vi "Dispatch PVMonitors.vi"(8 "Error In":errorcluster, 10 "PV Names (empty)":string[](array[string]), 11 "CS++GUIActor in":refnum<class "CS++GUIActor.lvclass">) -> (0 "Error Out":errorcluster, 3 "CS++GUIActor out":refnum<class "CS++GUIActor.lvclass">)   [LabVIEW 2015, in "CS++GUIActor.lvlib" / "CS++GUIActor.lvclass"]
doc: "Dispatch nested PVMonitor actors according to PV protocoll prefix."
uses:
  CS++GUIActor.lvclass
  CS++GUIActor Messages/Update-PV Msg/Update-PV Msg.lvclass
  CS++PVMonitor/CS++PVMonitor.lvclass
  CS++PVMonitor Messages/CS++PVUpdate Msg/CS++PVUpdate Msg.lvclass/CS++PVUpdate Msg.ctl
  CS++BaseActor/CS++BaseActor.lvclass/CS++BaseActor.ctl
  CS++GUIActor.lvclass/CS++GUIActor.ctl
  <vilib>/ActorFramework/Actor/Actor.lvclass/Actor.ctl
  <vilib>/ActorFramework/Message Enqueuer/Message Enqueuer.lvclass/Message Enqueuer.ctl
  Classes/CS++ProcessVariables/ProcessVariable/PV.lvclass/PV.ctl
  CS++PVMonitor/CS++PVMonitor.lvclass/CS++PVMonitor.ctl
  CS++PVMonitor Messages/Register PVs Msg/Register PVs Msg.lvclass/Register PVs Msg.ctl
  CS++BaseActor/Read Object Name.vi
  CS++BaseActor/Read CS++Factory.vi
  Read Associated Actor Name.vi
  <vilib>/ActorFramework/Message Enqueuer/Init from Existing Queue.vi
  <vilib>/ActorFramework/Message Enqueuer/Enqueue.vi
  <vilib>/ActorFramework/Message Priority Queue/Priority Enqueue.vi
  Classes/CS++ProcessVariables/ProcessVariable/PV.lvclass
  Classes/CS++BaseClasses/Factory/CS++Factory.lvclass
  <vilib>/ActorFramework/Message Enqueuer/Message Enqueuer.lvclass
  CS++PVMonitor Messages/Register PVs Msg/Register PVs Msg.lvclass
  <vilib>/ActorFramework/Actor/Actor.lvclass
  CS++BaseActor/CS++BaseActor.lvclass
  CS++PVMonitor Messages/CS++PVUpdate Msg/CS++PVUpdate Msg.lvclass
  Libraries/Base/CS++Base.lvlib
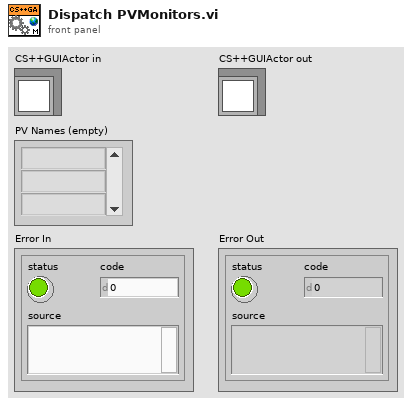
[diagram p1: front panel]
types:
  T1 = cluster{"Msgs":refnum<class "Update-PV Msg.lvclass">[]}[]
  T2 = cluster{"Msgs":refnum<class "Update-PV Msg.lvclass">[]}
  T3 = cluster{"Self Enqueuer":refnum<class "Message Enqueuer.lvclass">, "Msgs":refnum<class "Update-PV Msg.lvclass">[]}
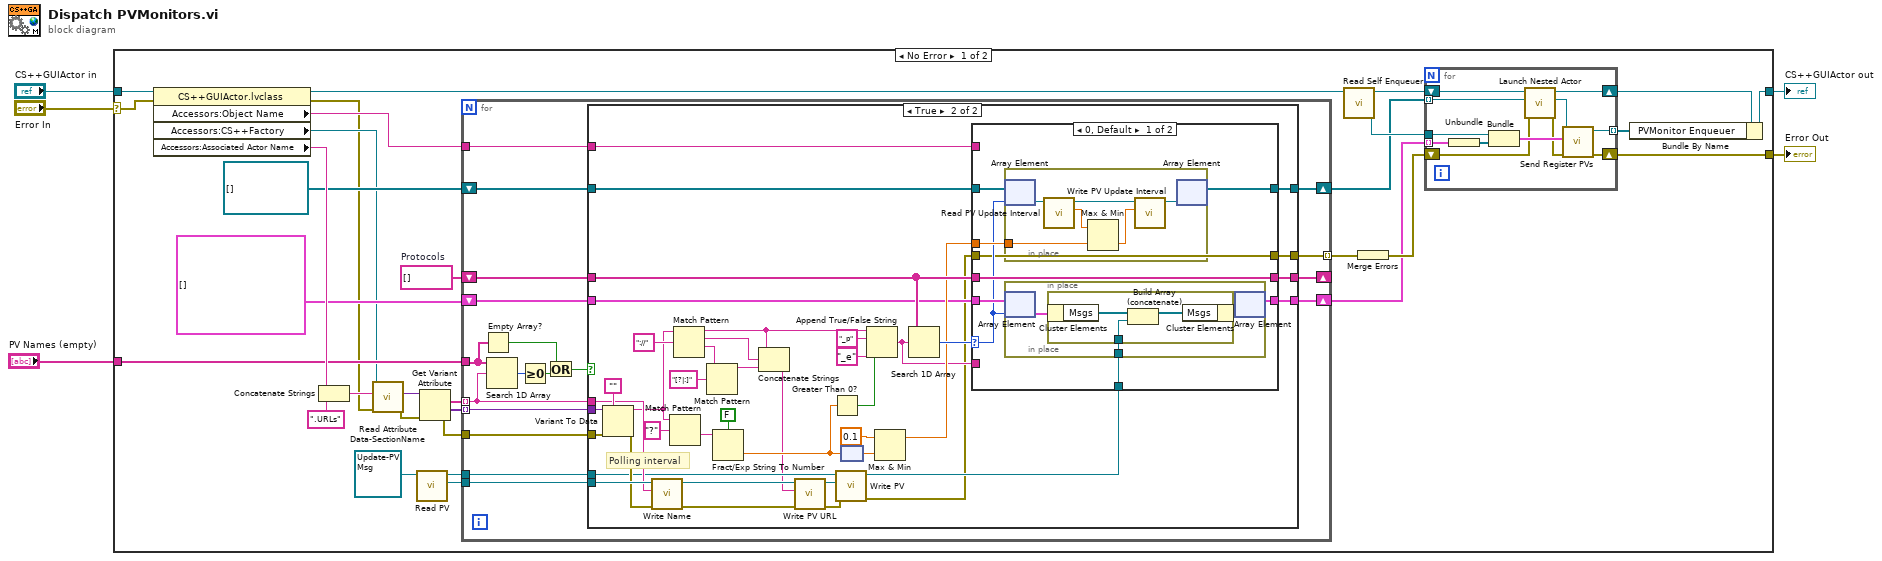
[diagram p0: block diagram]
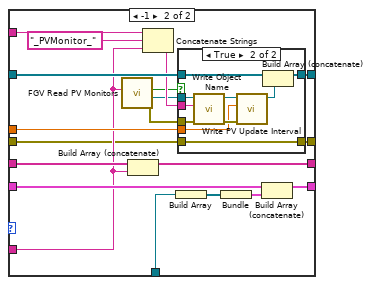
[diagram p3: hidden frame]
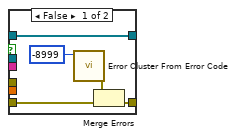
[diagram p4: hidden frame]
diagram:
  n1 = case shown="No Error" "Error In" {
    selector: "Error In" -> [w21 w167]
    tunnel: [w22 w167] -> w4
    tunnel: [w23 w166] -> w2
    tunnel: "CS++GUIActor in" -> [w24 w166]
    tunnel: "PV Names (empty)" -> [w12 _]
    frame No Error {
      w18 = string[] []  # Protocols
      n2 = property class="CS++GUIActor.lvclass"(reference=w24, error in=w21) -> (reference out=w25:refnum<class "CS++GUIActor.lvclass">, error out=w7:errorcluster, "Accessors:Object Name"=w17:string, "Accessors:CS++Factory"=w9:refnum<class "CS++Factory.lvclass">, "Accessors:Associated Actor Name"=w31:string)
      n3 = Concatenate Strings(w31, ".URLs" ("string")) -> (w8:string)
      n4 = call-dynamic "Read Attribute Data-SectionName.vi"("error in (no error)"=w7, "Object Name"=w8, "CS++Factory in"=w9) -> ("error out"=w11:errorcluster, "Attribute Data"=w10:variant)  [unwired: 6 in, 1 out]
      n5 = call "Read PV.vi"("CS++PVUpdate Msg in"=refnum<class "Update-PV Msg.lvclass"> refnum ("CS++DeviceGUIActor.lvlib:Update PV.lvclass")) -> ("PV"=w26:refnum<class "PV.lvclass">, "CS++PVUpdate Msg out"=w27:refnum<class "Update-PV Msg.lvclass">)  [unwired: 8 in, 1 out]
      n6 = Get Variant Attribute(Variant=w10, error in=w11) -> (names=w29:string[], values=w32:variant[], error out=w33:errorcluster)  [unwired: 2 in, 1 out]
      n7 = for {
        tunnel: w32 -> [w65] mode=indexing
        tunnel: w33 -> [w64]
        tunnel: w27 -> [w62]
        tunnel: w29 -> [w54] mode=indexing
        tunnel: w26 -> [w63]
        shift-right: [w61] -> w16
        shift-left: refnum<class "CS++PVMonitor.lvclass">[] [] -> [w58]
        shift-right: [w60] -> _
        shift-left: w18 -> [w59]
        tunnel: w17 -> [w57]
        shift-right: [w55] -> w13
        shift-left: T1 [] -> [w56]
        tunnel: w12 -> [w53]
        tunnel: [w48] -> w6 mode=indexing
        n8 = Empty Array?(array=w53) -> (empty?=w49:bool)
        n9 = Search 1D Array(1D array=w53, element=w54) -> (index of element=w51:i32)  [unwired: 1 in]
        n10 = Greater Or Equal To 0?(x=w51) -> (x >= 0?=w52:bool)
        n11 = Or(x=w49, y=w52) -> (x .or. y?=w50:bool)
        n12 = case shown="True" w50 {
          tunnel: w65 -> [_ w110]
          tunnel: w64 -> [w66 w109]
          tunnel: w63 -> [_ w107]
          tunnel: w54 -> [_ w106]
          tunnel: w62 -> [_ w104]
          tunnel: [w69 w95] -> w61
          tunnel: [w68 w94] -> w60
          tunnel: w59 -> [w68 w92]
          tunnel: w58 -> [w69 w91]
          tunnel: w57 -> [_ w86]
          tunnel: w56 -> [w67 w85]
          tunnel: [w67 w84] -> w55
          tunnel: [w66 w77] -> w48
          frame False {
          }
          frame True {
            # "Polling interval"
            n13 = Variant To Data(error in=w109, type="", Variant=w110) -> (data=w74:string, error out=w105:errorcluster)
            n14 = call "Write Name.vi"("error in (no error)"=w105, "Name"=w106, "PV in"=w107) -> ("error out"=w99:errorcluster, "PV out"=w100:refnum<class "PV.lvclass">)  [unwired: 7 in]
            n15 = Match Pattern(string=w74, regular expression="?" ("search string/char (-)")) -> (after substring=w102:string)  [unwired: 1 in, 3 out]
            n16 = Match Pattern(string=w74, regular expression="://") -> (before substring=w71:string, match substring=w70:string, after substring=w73:string)  [unwired: 1 in, 1 out]
            n17 = Match Pattern(string=w73, regular expression="[?|:]") -> (before substring=w75:string)  [unwired: 1 in, 3 out]
            n18 = Fract/Exp String To Number(use system decimal point (T)=FALSE, string=w102) -> (number=w88:dbl)  [unwired: 2 in, 1 out]
            n19 = Concatenate Strings(w71, w70, w75) -> (w72:string)
            n20 = call "Write PV URL.vi"("error in (no error)"=w99, "PV URL"=w72, "PV in"=w100) -> ("error out"=w97:errorcluster, "PV out"=w98:refnum<class "PV.lvclass">)  [unwired: 7 in]
            n21 = Greater Than 0?(x=w88) -> (x > 0?=w82:bool)
            n22 = call "Write PV.vi"("error in (no error)"=w97, "PV"=w98, "CS++PVUpdate Msg in"=w104) -> ("error out"=w78:errorcluster, "CS++PVUpdate Msg out"=w79:refnum<class "Update-PV Msg.lvclass">)  [unwired: 7 in]
            n23 = node(w88) -> (w90:dbl[unit])
            n24 = Append True/False String(1:w82, 2:"_e" ("false string"), 3:"_p" ("true string"), 4:w71) -> (0:w83:string)
            n25 = Max & Min(x=dbl[unit] 0.1, y=w90) -> (max(x,y)=w87:dbl[unit])  [unwired: 1 out]
            n26 = Search 1D Array(1D array=w92, element=w83) -> (index of element=w93:i32)  [unwired: 1 in]
            n27 = case shown="0, Default" w93 {
              selector: w93 -> [w114 _]
              tunnel: [w117 w150] -> w95
              tunnel: [w119 w149] -> w94
              tunnel: w83 -> [_ w137]
              tunnel: w92 -> [w119 w148]
              tunnel: w91 -> [w118 w147]
              tunnel: w87 -> [w116 w144]
              tunnel: w86 -> [_ w143]
              tunnel: w79 -> [w113 w142]
              tunnel: w85 -> [w115 w140]
              tunnel: [w112 w138] -> w84
              tunnel: w78 -> [w111 w134]
              tunnel: [w111 w132] -> w77
              frame 0, Default {
                n28 = in-place {
                  in-place-border: w116 -> [w131]
                  n29 = in-place-array #1(w118, w114) -> (w130:refnum<class "CS++PVMonitor.lvclass">)
                  n30 = call "Read PV Update Interval.vi"("CS++PVMonitor in"=w130) -> ("PV Update Interval"=w129:dbl[unit], "CS++PVMonitor out"=w128:refnum<class "CS++PVMonitor.lvclass">)  [unwired: 8 in, 1 out]
                  n31 = Max & Min(x=w129, y=w131) -> (min(x,y)=w126:dbl[unit])  [unwired: 1 out]
                  n32 = call "Write PV Update Interval.vi"("PV Update Interval"=w126, "CS++PVMonitor in"=w128) -> ("CS++PVMonitor out"=w127:refnum<class "CS++PVMonitor.lvclass">)  [unwired: 8 in, 1 out]
                  n33 = in-place-array #1(w127) -> (w117:refnum<class "CS++PVMonitor.lvclass">[])  [unwired: 1 out]
                }
                n34 = in-place {
                  in-place-border: w113 -> [w120]
                  n35 = in-place-array #2(w115, w114) -> (w122:T2)
                  n36 = in-place {
                    in-place-border: w120 -> [w124]
                    n37 = in-place-cluster #3(w122) -> ("Msgs"=w125:refnum<class "Update-PV Msg.lvclass">[])
                    n38 = Build Array (concatenate)(w125, w124) -> (w123:refnum<class "Update-PV Msg.lvclass">[])
                    n39 = in-place-cluster #3("Msgs"=w123) -> (w121:T2)
                  }
                  n40 = in-place-array #2(w121) -> (w112:T1)  [unwired: 1 out]
                }
              }
              frame -1 {
                n41 = call "FGV Read PV Monitors.vi"("PV Monitor"=w137) -> ("Error Out"=w135:errorcluster, "CS++PVMonitor"=w136:refnum<class "CS++PVMonitor.lvclass">, "Success"=w133:bool)  [unwired: 6 in, 2 out]
                n42 = Build Array (concatenate)(w148, w137) -> (w149:string[])
                n43 = Concatenate Strings(w143, "_PVMonitor_" ("Object Name"), w137) -> (w145:string)
                n44 = Build Array(w142) -> (w141:refnum<class "Update-PV Msg.lvclass">[])
                n45 = case shown="True" w133 {
                  tunnel: [w155 w165] -> w150
                  tunnel: w147 -> [w155 w164]
                  tunnel: w145 -> [_ w163]
                  tunnel: w144 -> [_ w157]
                  tunnel: w136 -> [_ w162]
                  tunnel: w135 -> [_ w161]
                  tunnel: w134 -> [w154 w160]
                  tunnel: [w153 w160] -> w132
                  frame False {
                    n46 = call <vilib>:"Error Cluster From Error Code.vi"("error code (0)"=-8999) -> ("error out"=w152:errorcluster)  [unwired: 8 in]
                    n47 = Merge Errors(w152, w154) -> (w153:errorcluster)
                  }
                  frame True {
                    n48 = call "Write Object Name.vi"("error in (no error)"=w161, "Object Name"=w163, "CS++BaseActor in"=w162) -> ("error out"=w158:errorcluster, "CS++BaseActor out"=w159:refnum<class "CS++PVMonitor.lvclass">)  [unwired: 7 in]
                    n49 = call "Write PV Update Interval.vi"("error in (no error)"=w158, "PV Update Interval"=w157, "CS++PVMonitor in"=w159) -> ("CS++PVMonitor out"=w156:refnum<class "CS++PVMonitor.lvclass">)  [unwired: 7 in, 1 out]
                    n50 = Build Array (concatenate)(w164, w156) -> (w165:refnum<class "CS++PVMonitor.lvclass">[])
                  }
                }
                n51 = Bundle(w141) -> (w139:cluster{refnum<class "Update-PV Msg.lvclass">[]})  [unwired: 1 in]
                n52 = Build Array (concatenate)(w140, w139) -> (w138:T1)
              }
            }
          }
        }
      }
      n53 = call <vilib>:"Read Self Enqueuer.vi"("Actor"=w25) -> ("Self Enqueuer"=w35:refnum<class "Message Enqueuer.lvclass">)  [unwired: 10 in]
      n54 = Merge Errors(w6) -> (w15:errorcluster)
      n55 = for {
        tunnel: w35 -> [w46]
        tunnel: w16 -> [w37] mode=indexing
        tunnel: w13 -> [w41] mode=indexing
        tunnel: [w38] -> w20 mode=indexing
        shift-right: [w39] -> w22
        shift-left: w15 -> [w43]
        shift-right: [w42] -> w30
        shift-left: w25 -> [w40]
        n56 = Unbundle(w41) -> ("Msgs"=w36:refnum<class "Update-PV Msg.lvclass">[])
        n57 = Bundle("Self Enqueuer"=w46, "Msgs"=w36) -> (w45:T3)  [unwired: 1 in]
        n58 = call <vilib>:"Launch Nested Actor.vi"("error in (no error)"=w43, "Nested Actor"=w37, "Caller Actor in"=w40) -> ("error out"=w44:errorcluster, "Nested Actor's Enqueuer"=w47:refnum<class "Message Enqueuer.lvclass">, "Caller Actor out"=w42:refnum<class "CS++GUIActor.lvclass">)  [unwired: 6 in]
        n59 = call "Send Register PVs.vi"("error in (no error)"=w44, "Register Info"=w45, "Message Enqueuer"=w47) -> ("error out"=w39:errorcluster, "Message Enqueuer out"=w38:refnum<class "Message Enqueuer.lvclass">)  [unwired: 7 in]
      }
      n60 = Bundle By Name(cluster=w30, "PVMonitor Enqueuer"=w20) -> (w23:refnum<class "CS++GUIActor.lvclass">)
    }
    frame Error {
    }
  }
  "Error Out" <- w4
  "CS++GUIActor out" <- w2
